vi "Handle Variable Header.vi"(8 "error in (no error)":errorcluster, 10 "Incoming Packets":u8[](array[numeric]) format="%08b", 11 "CONNECT in":refnum<class "CONNECT.lvclass">) -> (0 "error out":errorcluster, 1 "Variable Header Complete?":bool=TRUE, 2 "Remaining Packets":u8[](array[numeric]) format="%08b", 3 "CONNECT out":refnum<class "CONNECT.lvclass">)   [LabVIEW 2013, in "MQTT_Control_Packets.lvlib" / "CONNECT.lvclass"]
uses:
  CONNECT.lvclass
  ControlPacket/ControlPacket.lvclass/ControlPacket.ctl
  ControlPacket/ControlPacket.lvclass
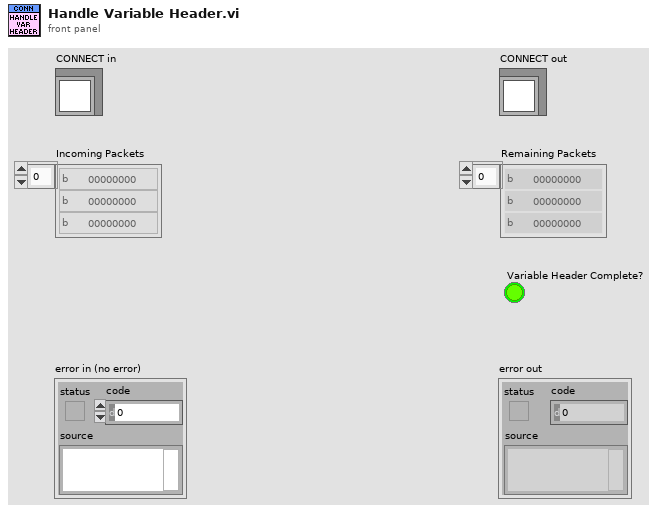
[diagram p1: front panel]
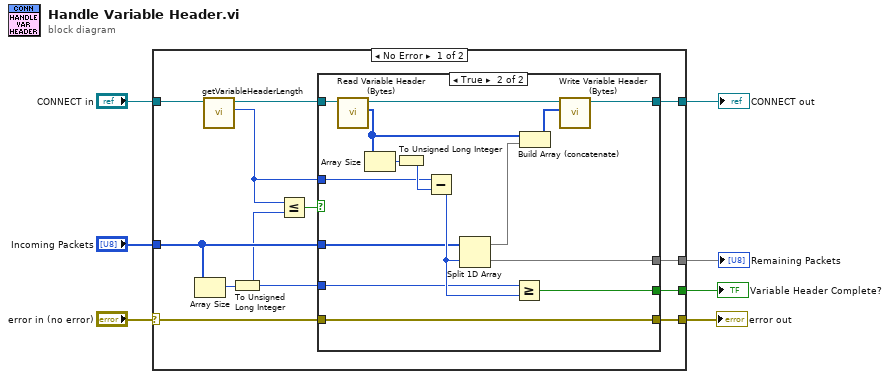
[diagram p0: block diagram]
diagram:
  n1 = case shown="No Error" "error in (no error)" {
    selector: "error in (no error)" -> [w8 w38]
    tunnel: "CONNECT in" -> [w19 w40]
    tunnel: "Incoming Packets" -> [w13 w39]
    tunnel: [w18 _] -> w5
    tunnel: [w17 w39] -> w4
    tunnel: [w16 w40] -> w3
    tunnel: [w9 w38] -> w1
    frame No Error {
      n2 = Array Size(array=w13) -> (size(s)=w14:i32)
      n3 = call-dynamic "getVariableHeaderLength.vi"("CONNECT in"=w19) -> ("VariableHeader size"=w11:u32, "CONNECT out"=w15:refnum<class "CONNECT.lvclass">)  [unwired: 8 in, 1 out]
      n4 = To Unsigned Long Integer(number=w14) -> (unsigned 32bit integer=w12:u32)
      n5 = Less Or Equal?(x=w11, y=w12) -> (x <= y?=w10:bool)
      n6 = case shown="True" w10 {
        tunnel: [_ w37] -> w18
        tunnel: [w21 w36] -> w17
        tunnel: [w22 w35] -> w16
        tunnel: w15 -> [w22 w34]
        tunnel: w13 -> [w21 w26]
        tunnel: w12 -> [_ w25]
        tunnel: w11 -> [_ w24]
        tunnel: [w20 w23] -> w9
        tunnel: w8 -> [w20 w23]
        frame False {
        }
        frame True {
          n7 = call "Read Variable Header (Bytes).vi"("ControlPacket in"=w34) -> ("Variable Header (Bytes)"=w31:u8[], "ControlPacket out"=w33:refnum<class "CONNECT.lvclass">)  [unwired: 9 in]
          n8 = Array Size(array=w31) -> (size(s)=w32:i32)
          n9 = To Unsigned Long Integer(number=w32) -> (unsigned 32bit integer=w28:u32)
          n10 = Subtract(x=w24, y=w28) -> (x-y=w27:u32)
          n11 = Split 1D Array(array=w26, index=w27) -> (first subarray=w30:u8[], second subarray=w36:u8[])
          n12 = Greater Or Equal?(x=w25, y=w27) -> (x >= y?=w37:bool)
          n13 = Build Array (concatenate)(w31, w30) -> (w29:u8[])
          n14 = call "Write Variable Header (Bytes).vi"("Variable Header (Bytes)"=w29, "ControlPacket in"=w33) -> ("ControlPacket out"=w35:refnum<class "CONNECT.lvclass">)  [unwired: 9 in]
        }
      }
    }
    frame Error {
    }
  }
  "error out" <- w1
  "CONNECT out" <- w3
  "Remaining Packets" <- w4
  "Variable Header Complete?" <- w5
